vi "Exp no 4b Full Adder.vi"() -> ()   [LabVIEW 2010]
panel:
  out "CARRY":bool
  out "SUM":bool
  in  "Z":bool
  in  "Y":bool
  in  "X":bool
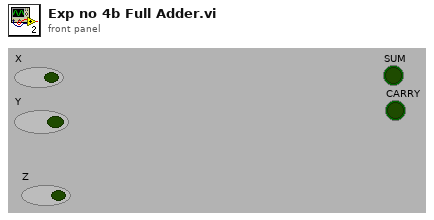
[diagram p1: front panel]
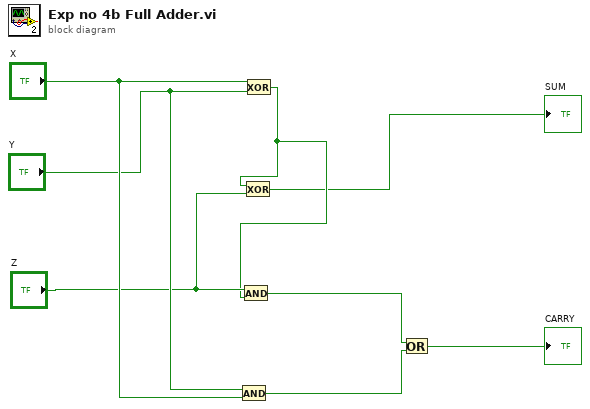
[diagram p0: block diagram]
diagram:
  n1 = And(x="Y", y="X") -> (x .and. y?=w1:bool)
  n2 = Exclusive Or(1:"Y", 2:"X") -> (0:w5:bool)
  n3 = And(x="Z", y=w5) -> (x .and. y?=w2:bool)
  n4 = Exclusive Or(1:"Z", 2:w5) -> (0:→"SUM":bool)
  n5 = Or(x=w2, y=w1) -> (x .or. y?=→"CARRY":bool)
